vi "System Log From Process Module.vi"(8 "error in":errorcluster, 10 "Socket Number":u16, 11 "Clear Error":bool) -> (0 "error out":errorcluster, 3 "SQL_Statement":string)   [LabVIEW 2023, in "HardwareAbstractionLayer_LVOOP.lvlib" / "Report.lvclass"]
uses:
  Report.lvclass
  Database/SQL Public VI/Control/DB Options.ctl
  Database/Database.lvclass
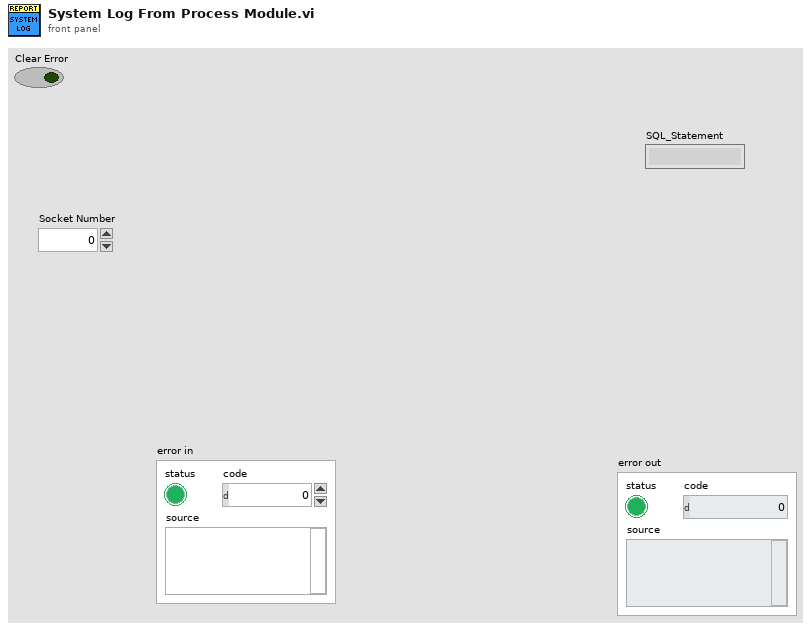
[diagram p1: front panel]
types:
  T1 = typedef "HardwareAbstractionLayer_LVOOP.lvlib/Database.lvclass/DB Options.ctl" = enum16{"Init", "Select Data", "Insert Data", "Update Data", "Delete Data", "Execute Query", "Create Schema", "Create Table", "List Tables", "List Columns", "Close"}
  T2 = typedef "HardwareAbstractionLayer_LVOOP.lvlib/Report.lvclass/Result FGV Data.ctl" = cluster{"Project Name":string, "Product Name":string, "Product Varient":string, "Test Name":string, "Test Phase":string, "Test Description":string, "Temp Chamber Name":string, "Schema":string, "Total No of Cycles":u32, "Current Cycle Number":u32, "Cycle Duration":u32, "Current Test Mode":string}
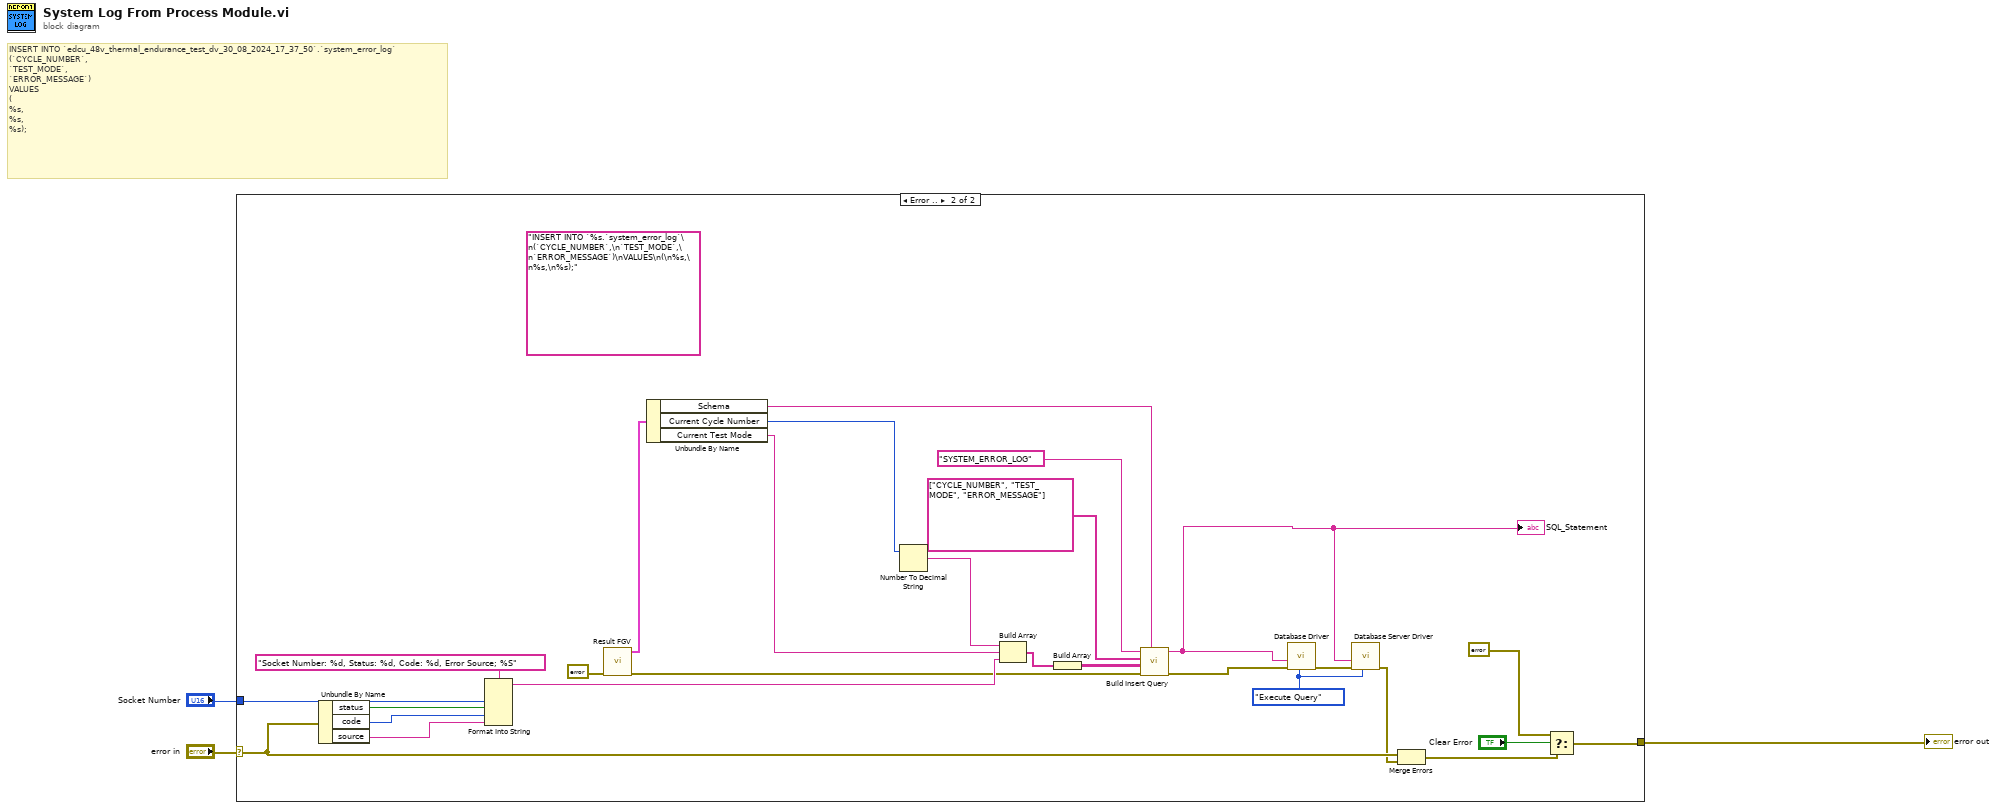
[diagram p0: block diagram]
diagram:
  # "INSERT INTO `edcu_48v_thermal_endurance_test_dv_30_08_2024_17_37_50`.`system_error_log`\n(`CYCLE_NUMBER`,\n`TEST_MODE`,\n`ERROR_MESSAGE`)\nVALUES\n(\n%s,\n%s,\n%s);"
  n1 = case shown="Error .." "error in" {
    selector: "error in" -> [w4 w16]
    tunnel: [w4 w15] -> w2
    tunnel: "Socket Number" -> [_ w6]
    frame No Error {
    }
    frame Error {
      w8 = DB_Options."Execute Query" ("Options")
      (unwired) "INSERT INTO `%s.`system_error_log`\n(`CYCLE_NUMBER`,\n`TEST_MODE`,\n`ERROR_MESSAGE`)\nVALUES\n(\n%s,\n%s,\n%s);"
      n2 = Unbundle By Name(w16) -> ("status"=w31:bool, "code"=w5:i32, "source"=w30:string)
      n3 = Format Into String(format string="Socket Number: %d, Status: %d, Code: %d, Error Source; %S", w6, w31, w5, w30) -> (resulting string=w22:string)  [unwired: 2 in, 1 out]
      n4 = call "Result FGV.vi"("error in"=errorcluster {"status"=FALSE, "code"=0, "source"=""}) -> ("error out"=w17:errorcluster, "Result FGV Data Out"=w28:T2)  [unwired: 9 in]
      n5 = Unbundle By Name(w28) -> ("Schema"=w26:string, "Current Cycle Number"=w20:u32, "Current Test Mode"=w21:string)
      n6 = Number To Decimal String(number=w20) -> (decimal integer string=w19:string)  [unwired: 1 in]
      n7 = Build Array(w19, w21, w22) -> (w25:string[])
      n8 = Build Array(w25) -> (w18:string[][])
      n9 = call "Build Insert Query.vi"("Schema Name"=w26, "error in (no error)"=w17, "Data"=w18, "Column Names"=string[] ["CYCLE_NUMBER", "TEST_MODE", "ERROR_MESSAGE"], "Table Name"="SYSTEM_ERROR_LOG") -> ("error out"=w10:errorcluster, "SQL"=w7:string)  [unwired: 5 in]
      "SQL_Statement" <- w7
      n10 = call "Database Driver.vi"("Options"=w8, "error in"=w10, "SQL query"=w7) -> ("error out"=w11:errorcluster)  [unwired: 5 in, 3 out]
      n11 = call "Database Server Driver.vi"("Options"=w8, "error in"=w11, "SQL query"=w7) -> ("error out"=w9:errorcluster)  [unwired: 5 in, 3 out]
      n12 = Merge Errors(w16, w9) -> (w12:errorcluster)
      n13 = Select(t=errorcluster {"status"=FALSE, "code"=0, "source"=""}, s="Clear Error", f=w12) -> (s? t:f=w15:errorcluster)
    }
  }
  "error out" <- w2
